vi "AutoScaleAmplitude.vi"(8 "error in (no error)":errorcluster, 9 "AutoScale":bool, 10 "Array":i16[](array[numeric]), 11 "Probe 1":i16) -> (0 "error out":errorcluster)   [LabVIEW 2018]
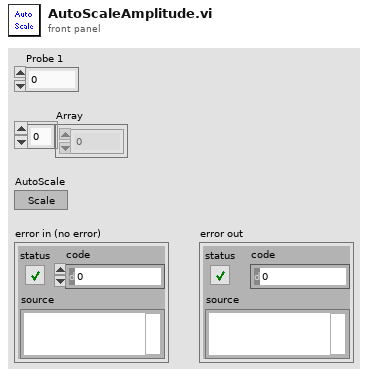
[diagram p1: front panel]
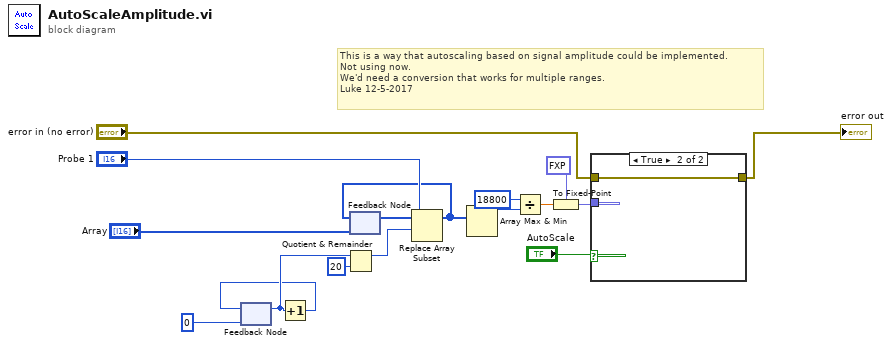
[diagram p0: block diagram]
diagram:
  # "This is a way that autoscaling based on signal amplitude could be implemented.\nNot using now. \nWe'd need a conversion that works for multiple ranges.\nLuke 12-5-2017"
  n1 = feedback #1(0 ("y")) -> (w13:i32)
  n2 = Increment(x=w13) -> (x+1=w12:i32)
  n3 = feedback-in #1(w12) -> ()
  n4 = Quotient & Remainder(x=w13, y=20) -> (x-y*floor(x/y)=w3:i32)  [unwired: 1 out]
  n5 = feedback #2("Array") -> (w2:i16[])
  n6 = Replace Array Subset(array=w2, new element="Probe 1", index=w3) -> (w7:i16[])
  n7 = feedback-in #2(w7) -> ()
  n8 = Array Max & Min(array=w7) -> (max value=w4:i16)  [unwired: 3 out]
  n9 = Divide(x=i16 18800, y=w4) -> (x/y=w6:dbl)
  n10 = To Fixed-Point(fixed-point type=fxp<+/-,23,23> 400.0 ("ScaleMeasurement"), number=w6) -> (fixed-point=w10:fxp<+/-,23,23>)
  n11 = case shown="True" "AutoScale" {
    tunnel: w10 -> [_ _]
    tunnel: [w18 w19] -> w15
    tunnel: "error in (no error)" -> [w18 w19]
    frame False {
    }
    frame True {
    }
  }
  "error out" <- w15
